vi "OAT Torsional Vibration (Digital Tacho) (Waveform) (N Ch - 1 Setting).vi"(0 "digital tacho info":T2[](array[typedef]), 2 "pulse/revolution (1)":i32=1 min=1, 4 "torsional vibration units":enum16{"RPM", "deg/s", "rad/s"}(ring), 5 "error in (no error)":errorcluster, 8 "reset? (F)":bool, 10 "compensate geometric imperfection? (F)":bool, 11 "output interval [s]":dbl=0.001 min=0.0) -> (14 "torsional vibration signals":waveform(dbl)[](array[waveform]), 15 "speed profiles":T1[](array[typedef]) {"speed [RPM]" format="%.2f"; "time [s]" format="%.2f"}, 18 "unit labels":string[](array[string]), 19 "error out":errorcluster)   [LabVIEW 2017, in "SoundVib_Torsional.lvlib"]
doc: "Calculates torsional vibration signals from digital tachometer signals. This VI can return torsional vibration signals as either waveform signals or even-angle signals. Wire data to the <B>digital tacho info</B> input to determine the polymorphic instance to use or manually select the instance."
uses:
  <vilib>/addons/Sound and Vibration/Order Analysis/Torsional Vibration/SoundVib_Torsional.lvlib
  <vilib>/addons/Sound and Vibration/Order Analysis/Tach Process/SubVIs/digital tach info.ctl
  <vilib>/addons/Sound and Vibration/Order Analysis/Tach Process/SubVIs/speed profile.ctl
  <vilib>/addons/Sound and Vibration/Order Analysis/Tach Process/SoundVib_TachProcess.lvlib
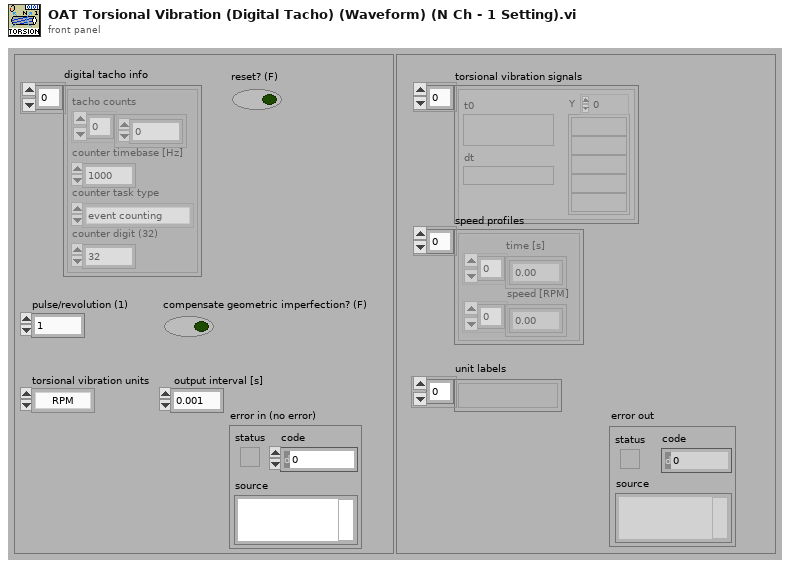
[diagram p1: front panel]
types:
  T1 = typedef "SoundVib_TachProcess.lvlib/speed profile.ctl" = cluster{"time [s]":dbl[], "speed [RPM]":dbl[]}
  T2 = typedef "SoundVib_TachProcess.lvlib/digital tach info.ctl" = cluster{"tacho counts":i64[], "counter timebase [Hz]":dbl, "counter task type":enum16{"period measurement", "event counting"}, "counter digit (32)":i32}
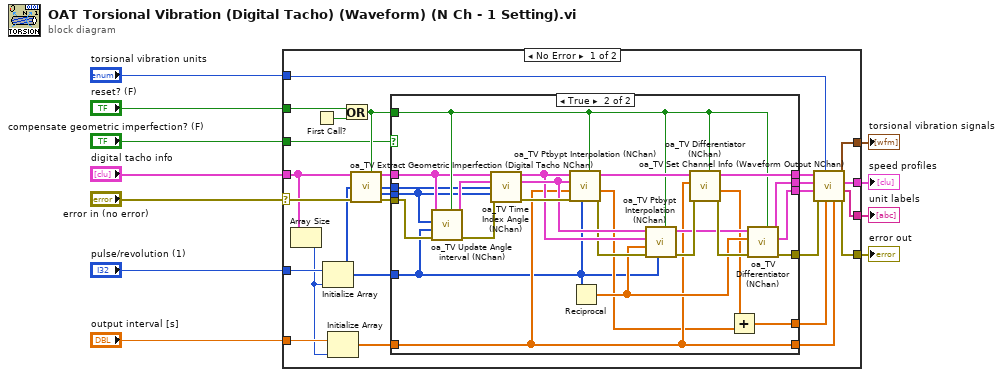
[diagram p0: block diagram]
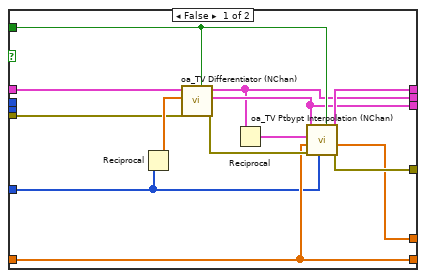
[diagram p2: hidden frame]
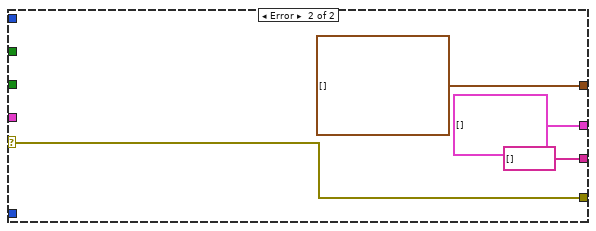
[diagram p3: hidden frame]
diagram:
  n1 = case shown="No Error" "error in (no error)" {
    selector: "error in (no error)" -> [w30 w79]
    tunnel: "compensate geometric imperfection? (F)" -> [w19 _]
    tunnel: "reset? (F)" -> [w34 _]
    tunnel: "digital tacho info" -> [w15 _]
    tunnel: "torsional vibration units" -> [w24 _]
    tunnel: [w25 waveform(dbl)[] []] -> w8
    tunnel: [w28 w79] -> w7
    tunnel: [w23 T1[] [] ("speed profile")] -> w5
    tunnel: [w18 string[] [] ("unit labels")] -> w3
    tunnel: "pulse/revolution (1)" -> [w17 _]
    tunnel: "output interval [s]" -> [w14 _]
    frame No Error {
      n2 = Array Size(array=w15) -> (size(s)=w13:i32)
      n3 = First Call?() -> (First Call?: T/F=w35:bool)
      n4 = Initialize Array(w17, w13) -> (w16:i32[])
      n5 = Initialize Array(w14, w13) -> (w12:dbl[])
      n6 = Or(x=w34, y=w35) -> (x .or. y?=w31:bool)
      n7 = call <vilib>:"oa_TV Extract Geometric Imperfection (Digital Tacho NChan).vi"("digital tacho info"=w15, "reset? (F)"=w31, "pulse/revolution"=w16, "error in (no error)"=w30) -> ("pulse positions"=w32:cluster{dbl[]}[], "revulotion"=w33:i32[], "revulotion index"=w36:i32[], "error out"=w37:errorcluster)  [unwired: 8 in]
      n8 = case shown="True" w19 {
        tunnel: w37 -> [w48 w54]
        tunnel: w36 -> [_ w53]
        tunnel: w33 -> [_ w55]
        tunnel: w32 -> [w50 w57]
        tunnel: w16 -> [w39 w52]
        tunnel: w31 -> [w47 w58]
        tunnel: [w41 w68] -> w29
        tunnel: [w46 w67] -> w27
        tunnel: [w38 w66] -> w26
        tunnel: [w40 w59] -> w22
        tunnel: w12 -> [w42 w62]
        tunnel: [w45 w63] -> w21
        tunnel: [w42 w62] -> w20
        frame False {
          n9 = Reciprocal(x=w39) -> (1/x=w49:dbl[])
          n10 = call <vilib>:"oa_TV Differentiator (NChan).vi"("reset? (False)"=w47, "error in (no error)"=w48, "delta X"=w49, "Y[n]"=w50) -> ("error out"=w43:errorcluster, "X[n]"=w45:cluster{dbl[]}[], "dY[n]/dX[n]"=w38:cluster{dbl[]}[])  [unwired: 4 in, 1 out]
          n11 = Reciprocal(x=w38) -> (1/x=w44:cluster{dbl[]}[])
          n12 = call <vilib>:"oa_TV Ptbypt Interpolation (NChan).vi"("reset? (F)"=w47, "buffer size"=w39, "error in (no error)"=w43, "dX"=w42, "Y"=w44, "X"=w45) -> ("error out"=w41:errorcluster, "X0"=w40:dbl[], "resampled Y"=w46:cluster{dbl[]}[])  [unwired: 2 in, 1 out]
        }
        frame True {
          n13 = call <vilib>:"oa_TV Update Angle interval (NChan).vi"("reset? (F)"=w58, "error in (no error)"=w54, "pulse/revolution"=w52, "revulotion index"=w53, "pulse position [s]"=w57) -> ("error out"=w51:errorcluster, "angle intervals"=w56:cluster{dbl[]}[])  [unwired: 5 in]
          n14 = call <vilib>:"oa_TV Time Index Angle (NChan).vi"("pulse positions"=w57, "angle intervals"=w56, "revulotion"=w55, "revulotion index"=w53, "error in (no error)"=w51) -> ("pulse positions"=w72:cluster{dbl[]}[], "angle"=w73:cluster{dbl[]}[], "error out"=w75:errorcluster)  [unwired: 8 in]
          n15 = call <vilib>:"oa_TV Ptbypt Interpolation (NChan).vi"("reset? (F)"=w58, "buffer size"=w52, "error in (no error)"=w75, "dX"=w62, "Y"=w73, "X"=w72) -> ("error out"=w71:errorcluster, "X0"=w60:dbl[], "resampled Y"=w74:cluster{dbl[]}[])  [unwired: 2 in, 1 out]
          n16 = Reciprocal(x=w52) -> (1/x=w65:dbl[])
          n17 = call <vilib>:"oa_TV Ptbypt Interpolation (NChan).vi"("reset? (F)"=w58, "buffer size"=w52, "error in (no error)"=w71, "dX"=w65, "Y"=w72, "X"=w73) -> ("error out"=w70:errorcluster, "resampled Y"=w64:cluster{dbl[]}[])  [unwired: 2 in, 2 out]
          n18 = call <vilib>:"oa_TV Differentiator (NChan).vi"("reset? (False)"=w58, "error in (no error)"=w70, "delta X"=w62, "Y[n]"=w74) -> ("error out"=w69:errorcluster, "Delay"=w61:dbl[], "dY[n]/dX[n]"=w67:cluster{dbl[]}[])  [unwired: 4 in, 1 out]
          n19 = Add(x=w61, y=w60) -> (x+y=w59:dbl[])
          n20 = call <vilib>:"oa_TV Differentiator (NChan).vi"("reset? (False)"=w58, "error in (no error)"=w69, "delta X"=w65, "Y[n]"=w64) -> ("error out"=w68:errorcluster, "X[n]"=w63:cluster{dbl[]}[], "dY[n]/dX[n]"=w66:cluster{dbl[]}[])  [unwired: 4 in, 1 out]
        }
      }
      n21 = call <vilib>:"oa_TV Set Channel Info (Waveform Output NChan).vi"("dt"=w20, "t0"=w22, "torisional vibration unit (RPM)"=w24, "error in (no error)"=w29, "pulse position"=w21, "seconds/revolution"=w26, "revolutions/minute"=w27) -> ("error out"=w28:errorcluster, "unit labels"=w18:string[], "speed profile"=w23:T1[], "torsional vibration"=w25:waveform(dbl)[])  [unwired: 1 in]
    }
    frame Error {
    }
  }
  "error out" <- w7
  "torsional vibration signals" <- w8
  "speed profiles" <- w5
  "unit labels" <- w3
